vi "Initialise.vi"() -> (2 "Pixel Data out":u32[][](array[numeric]), 3 "Scene out":refnum<class "Scene.lvclass">)   [LabVIEW 2020, in "Benchmark.lvlib"]
uses:
  Benchmark.lvlib
  Scene/Scene.lvclass
  Libraries/Raster/Raster.lvlib
  Libraries/Raster/Rectangle Dimensions.ctl
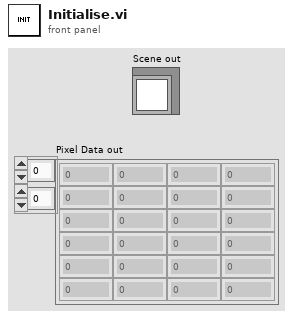
[diagram p1: front panel]
types:
  T1 = typedef "Raster.lvlib/Rectangle Dimensions.ctl" = cluster{"Width":u32, "Height":u32}
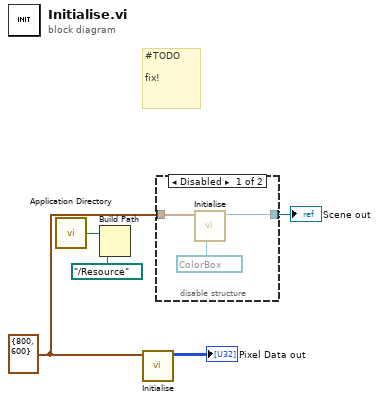
[diagram p0: block diagram]
diagram:
  w5 = T1 {"Width"=800, "Height"=600} ("Screen Dimensions")
  # "#TODO\n\nfix!"
  n1 = call <vilib>:"Application Directory.vi"() -> ("Application Directory"=w3:path)
  n2 = Build Path(base path=w3, name or relative path=path "../Resource") -> ()  [unwired: 1 out]
  n3 = call "Initialise.vi"("Screen Dimensions"=w5) -> ("Pixel Data out"=→"Pixel Data out":u32[][])  [unwired: 10 in]
  n4 = disable-structure shown="Disabled" {
    disable-tunnel: w5 -> [w8 _]
    disable-tunnel: [w6 _] -> w2
    frame Disabled {
      n5 = call "Initialise.vi"("Diffuse Colour"=refnum<vi> refnum, "Screen Dimensions"=w8) -> ("Scene out"=w6:refnum<class "Scene.lvclass">)  [unwired: 8 in, 1 out]
    }
    frame Enabled {
    }
  }
  "Scene out" <- w2
